vi "noise_eater.vi"(0 "In val":i16, 1 "AO cluster":T4, 2 "NE cluster":T3) -> (7 "Out val":i16)   [LabVIEW 2019]
uses:
  <vilib>/addons/control/pid/fpga.llb/XNode/niFpgaPID.xnode
  <vilib>/eio/EIONode/EIONode.xnode
  <vilib>/rvi/eio/common/nirviEmuTemplateMethod_errors.vi
  <vilib>/Platform/TimedLoop/XDataNode/wakeup.ctl
  <vilib>/Platform/TimedLoop/XDataNode/XDNodeRunTimeDep.lvlib
  <vilib>/Platform/TimedLoop/XDataNode/nitl_modes.ctl
  <vilib>/Platform/TimedLoop/XDataNode/timing_clust.ctl
  <vilib>/Platform/TimedLoop/XDataNode/XDataNode.xnode
panel:
  out "Input Signal / mV":fxp<+/-,19,14> format="%.3g"
  in  "AO4 max":i16 min=0 max=3277
  out "AO4":bool
  out "AO4 on":i16
  out "AO4 off":i16
  out "override noise eater?":bool
  out "Setpoint (H)":fxp<+/-,16,16>
  out "Control Signal / mV":fxp<+/-,19,14> format="%.3g"
  out "Control Signal":i16(graph)
  out "Setpoint (L)":fxp<+/-,16,16> format="%.3f"
  in  "Reinitialise controller":bool
  out "PID gains":T1={"Proportional gain Kc"=0.0, "Integral time Ti [min]"=2.0, "Derivative time Td [min]"=0.0}
  out "Controller output range":T2={"Output high"=10.0, "Output low"=-10.0}
  in  "High power":bool
  in  "start sequence":bool
  in  "AOM":bool
  out "Seq DO bits":u64
  out "Seq AO bits":u8
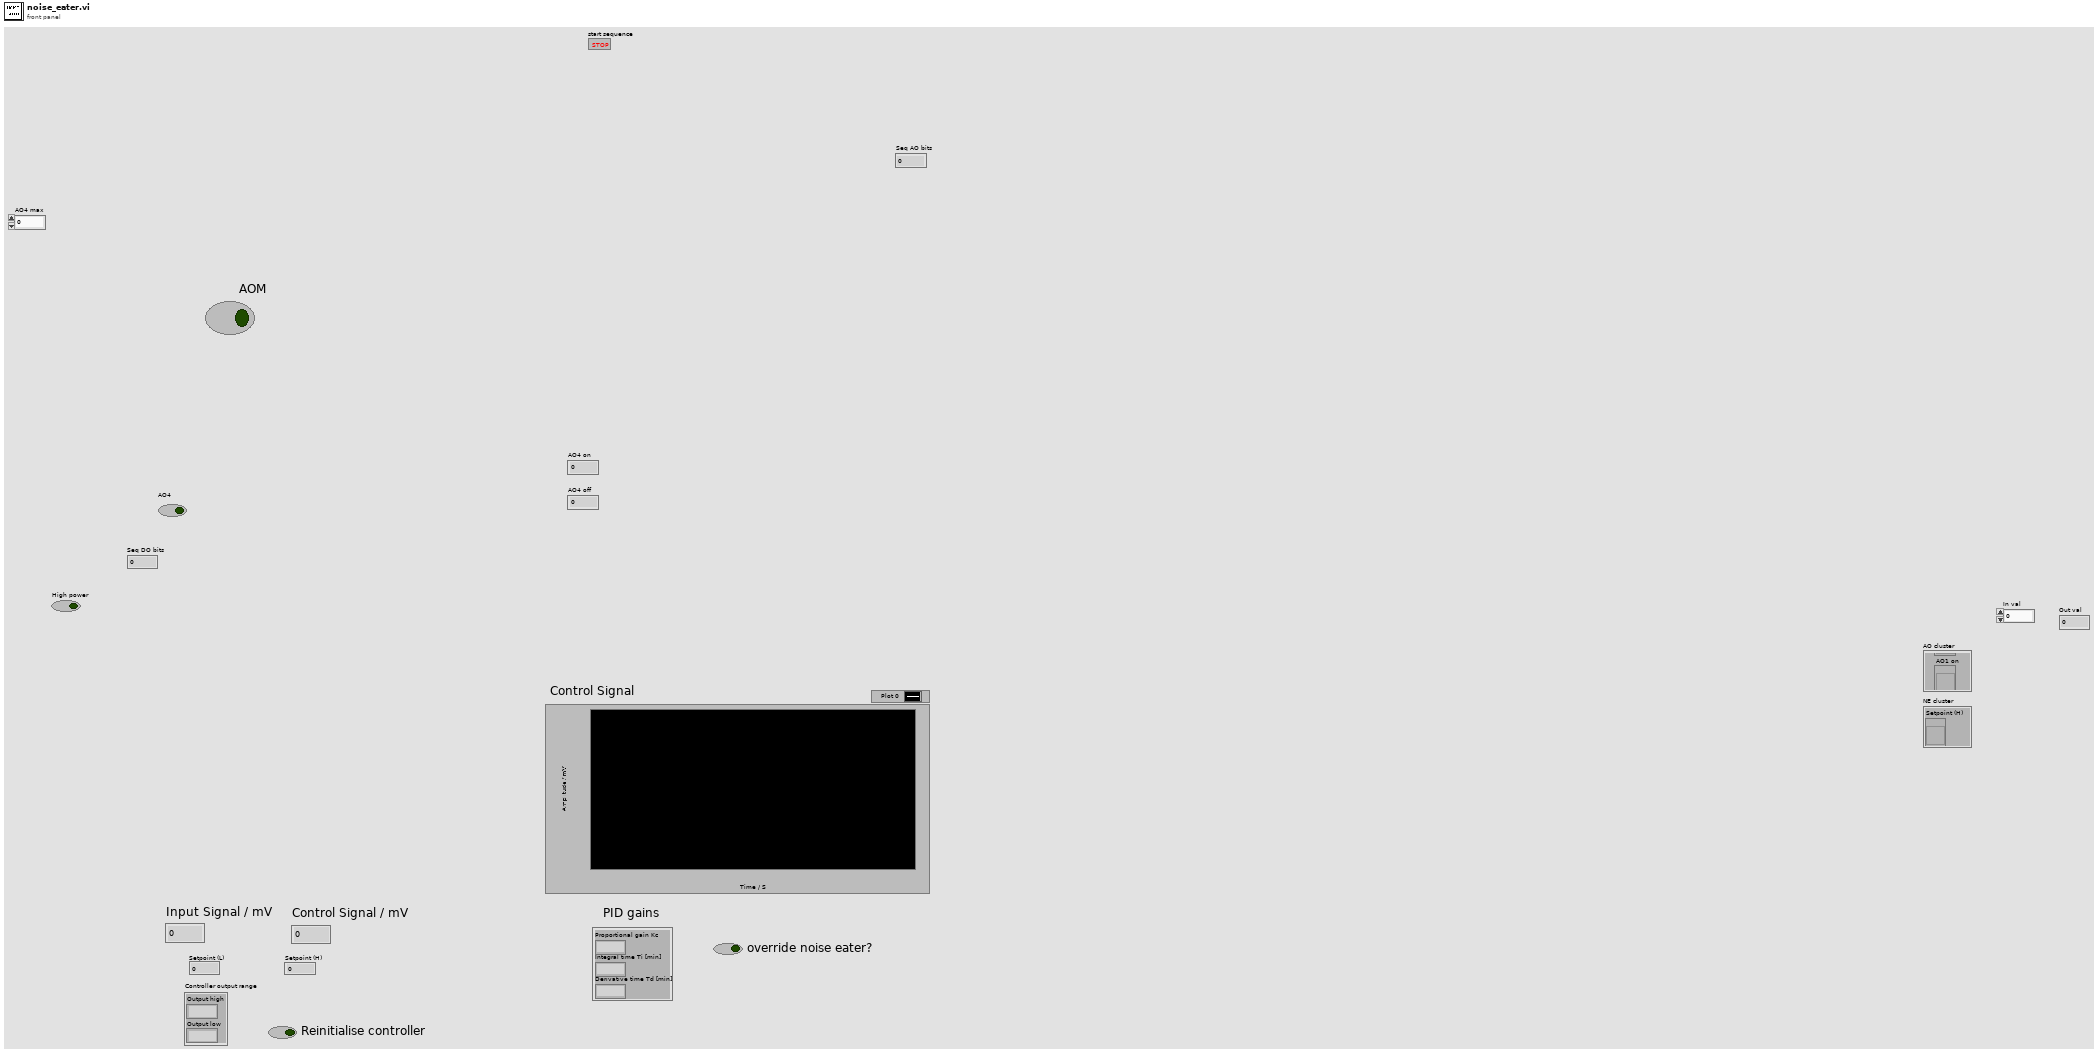
[diagram p1: front panel]
types:
  T1 = cluster{"Proportional gain Kc":fxp<+/-,16,8>, "Integral time Ti [min]":fxp<+/-,16,8>, "Derivative time Td [min]":fxp<+/-,16,8>}
  T2 = cluster{"Output high":fxp<+/-,16,16>, "Output low":fxp<+/-,16,16>}
  T3 = cluster{"Setpoint (H)":refnum<vi>, "Setpoint (L)":refnum<vi>, "Control Signal / mV":refnum<vi>, "Input Signal / mV":refnum<vi>, "Filtered Input 2":refnum<vi>, "override noise eater?":refnum<vi>, "High power":refnum<vi>, "Controller output range":refnum<vi>, "PID gains":refnum<vi>, "Filtered Input":refnum<vi>, "Control Signal":refnum<vi>}
  T4 = cluster{"AO1":refnum<vi>, "AO2":refnum<vi>, "AO3":refnum<vi>, "AO4":refnum<vi>, "AO1 on":refnum<vi>, "AO1 off":refnum<vi>, "AO2 on":refnum<vi>, "AO2 off":refnum<vi>, "AO3 on":refnum<vi>, "AO3 off":refnum<vi>, "AO4 on":refnum<vi>, "AO4 off":refnum<vi>, "AO5":refnum<vi>, "AO6":refnum<vi>, "AO7":refnum<vi>}
  T5 = typedef "XDNodeRunTimeDep.lvlib/timing_clust.ctl" = cluster{"Expected End [f-1]":u64, "Actual End [f-1]":u64, "Finished Late? [f-1]":bool, "Expected End [i-1]":u64, "Actual End [i-1]":u64, "Finished Late? [i-1]":bool, "Expected Start [i]":u64, "Actual Start [i]":u64, "Expected Start [f]":u64, "Actual Start [f]":u64, "Source Name":string, "Structure Name":string, "Period":i64, "Deadline":i64, "Offset":i64, "Start":i64, "Priority":i32, "Timeout":i32, "Mode":T6, "Wakeup Reason":T7, "Error":errorcluster, "Source Type":string, "Secondary Source Type":string, "Global End Time":u64, "Global Start Time":u64, "Frame Duration":u64, "Iteration Duration":u64, "Assigned CPU":i32, "I/O Scan Engine Mode":u32}
  T6 = typedef "XDNodeRunTimeDep.lvlib/nitl_modes.ctl" = enum32{"No Change", "Process missed periods, maintain original phase", "Discard missed periods, maintain original phase", "Process missed periods, ignore original phase", "Discard missed periods, ignore original phase"}
  T7 = typedef "XDNodeRunTimeDep.lvlib/wakeup.ctl" = enum32{"Normal", "Aborted", "Asynchronous wakeup", "Timing source error", "Timed loop error", "Timeout"}
  T8 = cluster{"proportional gain (Kc)":i16, "integral gain (Kc*Ts/Ti)":i16, "derivative gain (Kc*Td/Ts)":i16}
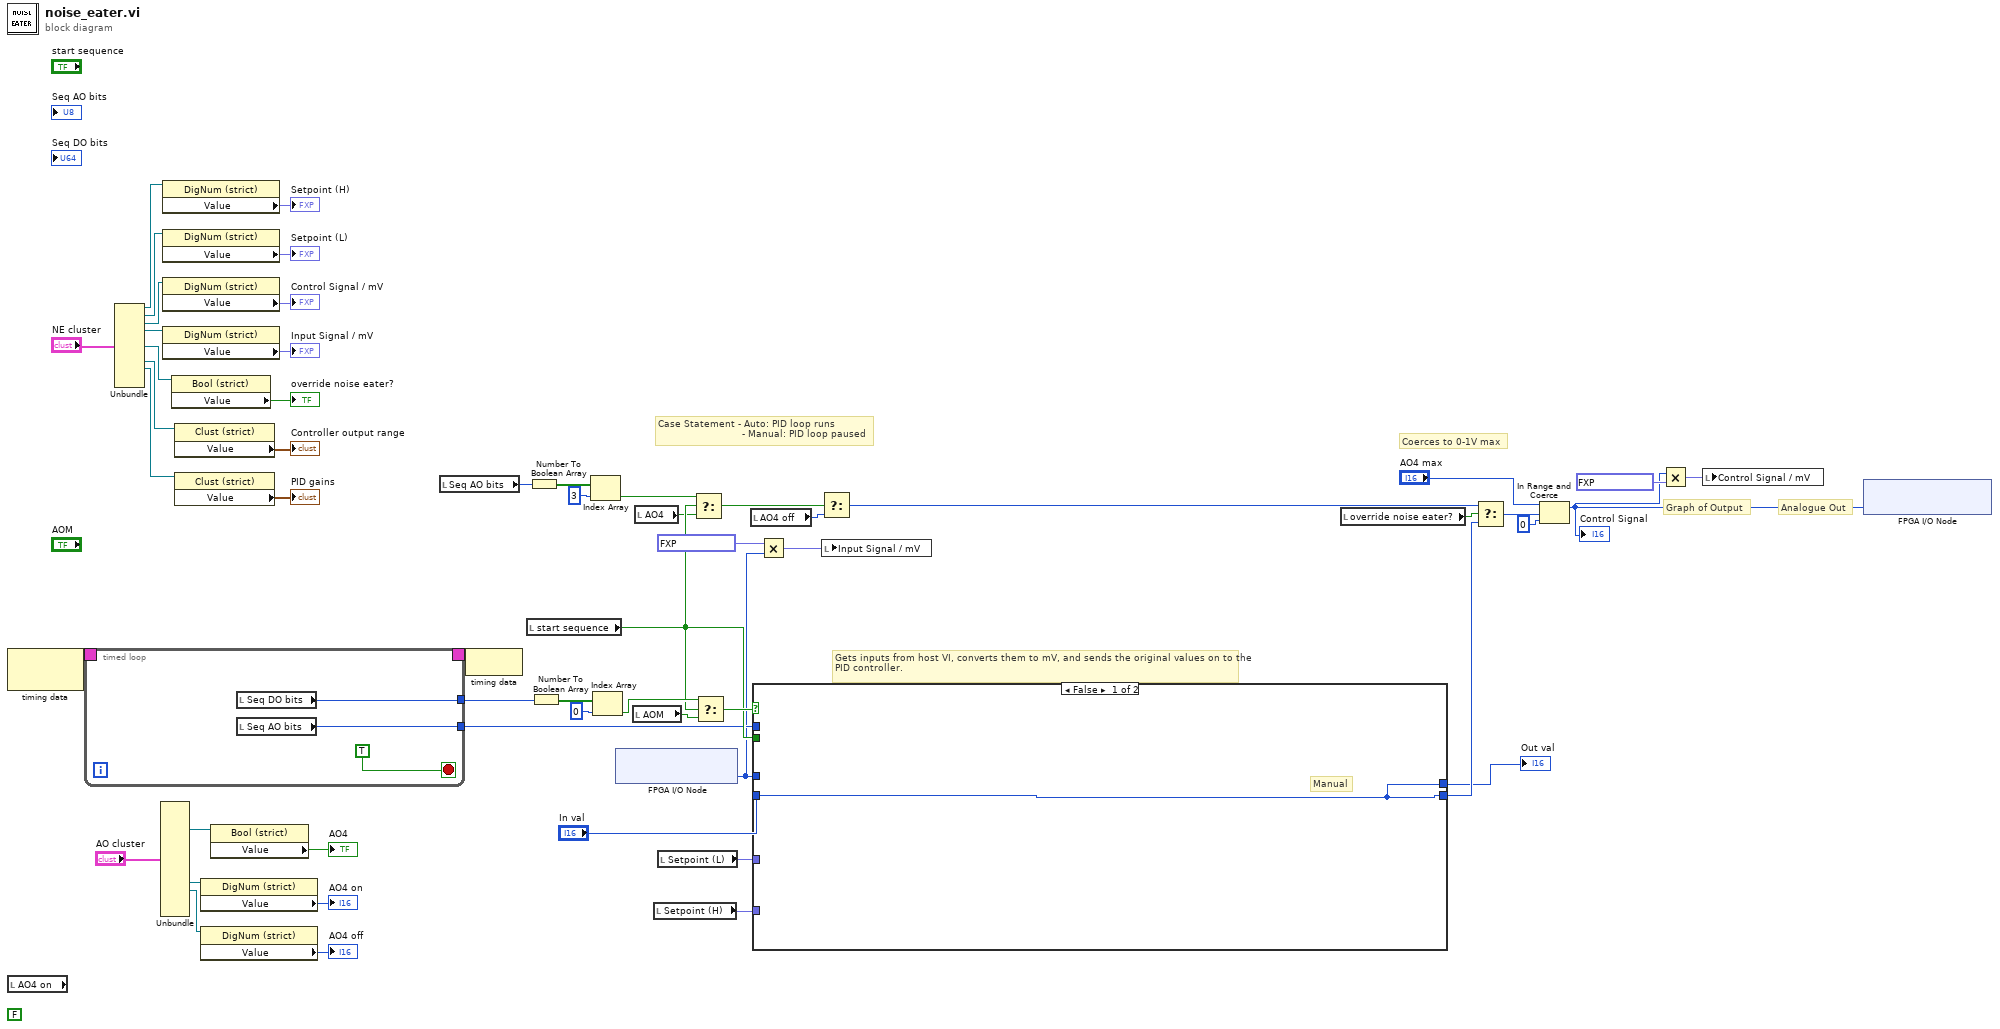
[diagram p0: block diagram]
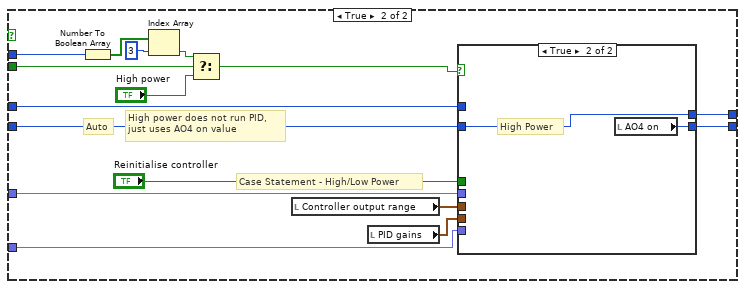
[diagram p2: hidden frame]
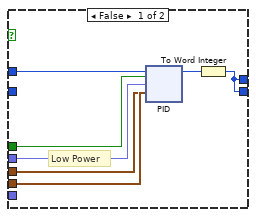
[diagram p3: hidden frame]
diagram:
  (unwired) FALSE
  # "Coerces to 0-1V max"
  # "Graph of Output"
  # "Gets inputs from host VI, converts them to mV, and sends the original values on to the PID controller."
  # "Case Statement - Auto: PID loop runs\n                            - Manual: PID loop paused"
  # "Analogue Out"
  n1 = node-c288() -> (w55:T5)  [unwired: 1 in]
  n2 = local read "AO4 on"() -> ()  [unwired: 1 out]
  n3 = timed-loop {
    timing: w55 -> [_]
    timing-out: [_] -> w54
    tunnel: [w58] -> w49
    tunnel: [w57] -> w38
    stop <- TRUE stop-if-true
    n4 = local read "Seq DO bits"() -> (w58:u64)
    n5 = local read "Seq AO bits"() -> (w57:u8)
  }
  n6 = Unbundle("NE cluster") -> ("Setpoint (H)"=w19:refnum<vi>, "Setpoint (L)"=w18:refnum<vi>, "Control Signal / mV"=w13:refnum<vi>, "Input Signal / mV"=w12:refnum<vi>, "override noise eater?"=w26:refnum<vi>, "Controller output range"=w22:refnum<vi>, "PID gains"=w23:refnum<vi>)  [unwired: 4 out]
  n7 = Unbundle("AO cluster") -> ("AO4"=w29:refnum<vi>, "AO4 on"=w7:refnum<vi>, "AO4 off"=w6:refnum<vi>)  [unwired: 12 out]
  n8 = property class="DigNum (strict)"(reference=w19) -> ("Value"=→"Setpoint (H)":fxp<+/-,16,16>)  [unwired: 1 in, 2 out]
  n9 = property class="DigNum (strict)"(reference=w18) -> ("Value"=→"Setpoint (L)":fxp<+/-,16,16>)  [unwired: 1 in, 2 out]
  n10 = property class="DigNum (strict)"(reference=w13) -> ("Value"=→"Control Signal / mV":fxp<+/-,19,14>)  [unwired: 1 in, 2 out]
  n11 = property class="DigNum (strict)"(reference=w12) -> ("Value"=→"Input Signal / mV":fxp<+/-,19,14>)  [unwired: 1 in, 2 out]
  n12 = property class="Bool (strict)"(reference=w26) -> ("Value"=→"override noise eater?":bool)  [unwired: 1 in, 2 out]
  n13 = property class="Clust (strict)"(reference=w22) -> ("Value"=→"Controller output range":T2)  [unwired: 1 in, 2 out]
  n14 = property class="Clust (strict)"(reference=w23) -> ("Value"=→"PID gains":T1)  [unwired: 1 in, 2 out]
  n15 = property class="DigNum (strict)"(reference=w7) -> ("Value"=→"AO4 on":i16)  [unwired: 1 in, 2 out]
  n16 = property class="DigNum (strict)"(reference=w6) -> ("Value"=→"AO4 off":i16)  [unwired: 1 in, 2 out]
  n17 = property class="Bool (strict)"(reference=w29) -> ("Value"=→"AO4":bool)  [unwired: 1 in, 2 out]
  n18 = local read "Seq AO bits"() -> (w43:u8)
  n19 = node-c288(w54) -> ()
  n20 = local read "start sequence"() -> (w39:bool)
  n21 = Number To Boolean Array(number=w43) -> (Boolean array=w44:bool[])
  n22 = Number To Boolean Array(number=w49) -> (Boolean array=w51:bool[])
  n23 = Index Array(array=w44, index=3) -> (element=w40:bool)
  n24 = Index Array(array=w51, index=0) -> (element=w46:bool)
  n25 = xnode "FPGA I/O Node"() -> ("Connector0/AI0"=w32:i16)  [unwired: 1 in, 1 out]
  n26 = local read "AOM"() -> (w48:bool)
  n27 = local read "AO4"() -> (w27:bool)
  n28 = local read "Setpoint (H)"() -> (w16:fxp<+/-,16,16>)
  n29 = local read "Setpoint (L)"() -> (w14:fxp<+/-,16,16>)
  n30 = Select(t=w40, s=w39, f=w27) -> (s? t:f=w41:bool)
  n31 = Select(t=w46, s=w39, f=w48) -> (s? t:f=w47:bool)
  n32 = local read "AO4 off"() -> (w3:i16)
  n33 = case shown="False" w47 {
    tunnel: [w61 w68] -> w52
    tunnel: w14 -> [_ w76]
    tunnel: w16 -> [_ w75]
    tunnel: w39 -> [_ w74]
    tunnel: w38 -> [_ w67]
    tunnel: [w61 w66] -> w1
    tunnel: "In val" -> [w61 w65]
    tunnel: w32 -> [_ w64]
    frame False {
      # "Manual"
    }
    frame True {
      # "High power does not run PID,\njust uses AO4 on value"
      # "Case Statement - High/Low Power"
      # "Auto"
      n34 = Number To Boolean Array(number=w67) -> (Boolean array=w70:bool[])
      n35 = Index Array(array=w70, index=3) -> (element=w69:bool)
      n36 = Select(t=w69, s=w74, f="High power") -> (s? t:f=w73:bool)
      n37 = local read "Controller output range"() -> (w62:T2)
      n38 = local read "PID gains"() -> (w63:T1)
      n39 = case shown="True" w73 {
        tunnel: "Reinitialise controller" -> [w82 _]
        tunnel: w63 -> [w84 _]
        tunnel: w62 -> [w83 _]
        tunnel: [w79 w114] -> w68
        tunnel: w76 -> [w81 _]
        tunnel: w75 -> [_ _]
        tunnel: [w79 w113] -> w66
        tunnel: w65 -> [_ w113]
        tunnel: w64 -> [w78 _]
        frame False {
          # "Low Power"
          n40 = xnode ("PID")("process variable"=w78, "reset?"=w82, "setpoint"=w81, "PID gains"=w84, "output range"=w83) -> ("output"=w80:i16)
          n41 = To Word Integer(number=w80) -> (16bit integer=w79:i16)
        }
        frame True {
          # "High Power"
          n42 = local read "AO4 on"() -> (w114:i16)
        }
      }
    }
  }
  "Out val" <- w1
  n43 = Multiply(x=fxp<+,10,-1> 0.30517578125, y=w32) -> (x*y=w10:fxp<+/-,26,15>)
  n44 = Select(s=w41, f=w3) -> (s? t:f=w42:i16)  [unwired: 1 in]
  n45 = local write "Input Signal / mV"(w10) -> ()
  n46 = local read "override noise eater?"() -> (w24:bool)
  n47 = Select(t=w42, s=w24, f=w52) -> (s? t:f=w36:i16)
  n48 = In Range and Coerce(upper limit="AO4 max", x=w36, lower limit=i16 0) -> (coerced(x)=w35:i16)  [unwired: 1 out]
  "Control Signal" <- w35
  n49 = Multiply(x=w35, y=fxp<+,10,-1> 0.30517578125) -> (x*y=w8:fxp<+/-,26,15>)
  n50 = local write "Control Signal / mV"(w8) -> ()
  n51 = xnode "FPGA I/O Node"("Connector0/AO4"=w35) -> ()  [unwired: 1 in, 1 out]
